vi "Sprinklernew.vi"() -> ()   [LabVIEW 2013]
doc: "This Vi is a simulation of Sprinkler system which service four zone\n-East\n-West\n-North\n-South\nIndicator on front panel indicate the zone that is currently running.\n\nThe controller loads the data to Zone Setup Array from .csv file.\n-It runs when user press start.\nWhen Run selector is at \nSingle position: the controller will serve each zone for the set timing and wait for input.\nContinuous Position: It will run contineously.\n\nSequence of operation: \nStart(Application): It will initialize all the controls and indicator to its default value.\nSetup: It will allow the user to change in Zone setup array.\nStart: It will start the VI.\nRain Sensor: Shows Rain in Status and indicators will not respond in this case."
uses:
  Controls/Sprinkler Cmd data cluster.ctl
  Controls/Sprinkler States.ctl
  SubVIs/water pressuer sensor fgv.ctl
  Controls/Read States.ctl
panel:
  in  "Zone Setup Array":cluster{"Zone Selector":string, "Timing":dbl}[](array[cluster])
  out "Controller Status":string
  out "Zone Indicators":T1
  in  "Water Pressure Sensor (%)":u32(slide) scale=0.0..100.0
  in  "Rain Sensor":bool
  in  "Run Selector":bool
  in  "Setup":bool
  in  "Start":bool
  in  "stop":bool
  # "Controls"
  # "Simulation Controls"
  # "Rain"
  # "No Rain"
  # "Continuous"
  # "Single"
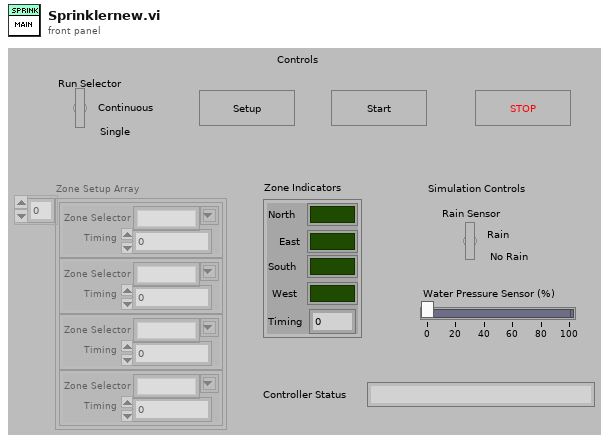
[diagram p1: front panel]
types:
  T1 = cluster{"North":bool, "East":bool, "South":bool, "West":bool, "Timing":u32}
  T2 = typedef "Sprinkler Cmd data cluster.ctl" = cluster{"Data":variant, "Command":T3}
  T3 = typedef "Sprinkler States.ctl" = enum16{"Initialize", "Setup", "Start", "Rain Sensor", "Stop"}
  T4 = typedef "water pressuer sensor fgv.ctl" = enum16{"Set data ", "Get data"}
  T5 = enum8{"Enabled", "Disabled", "Disabled and Grayed Out"}
  T6 = typedef "Read States.ctl" = enum16{"Initialize ", "Read", "Stop"}
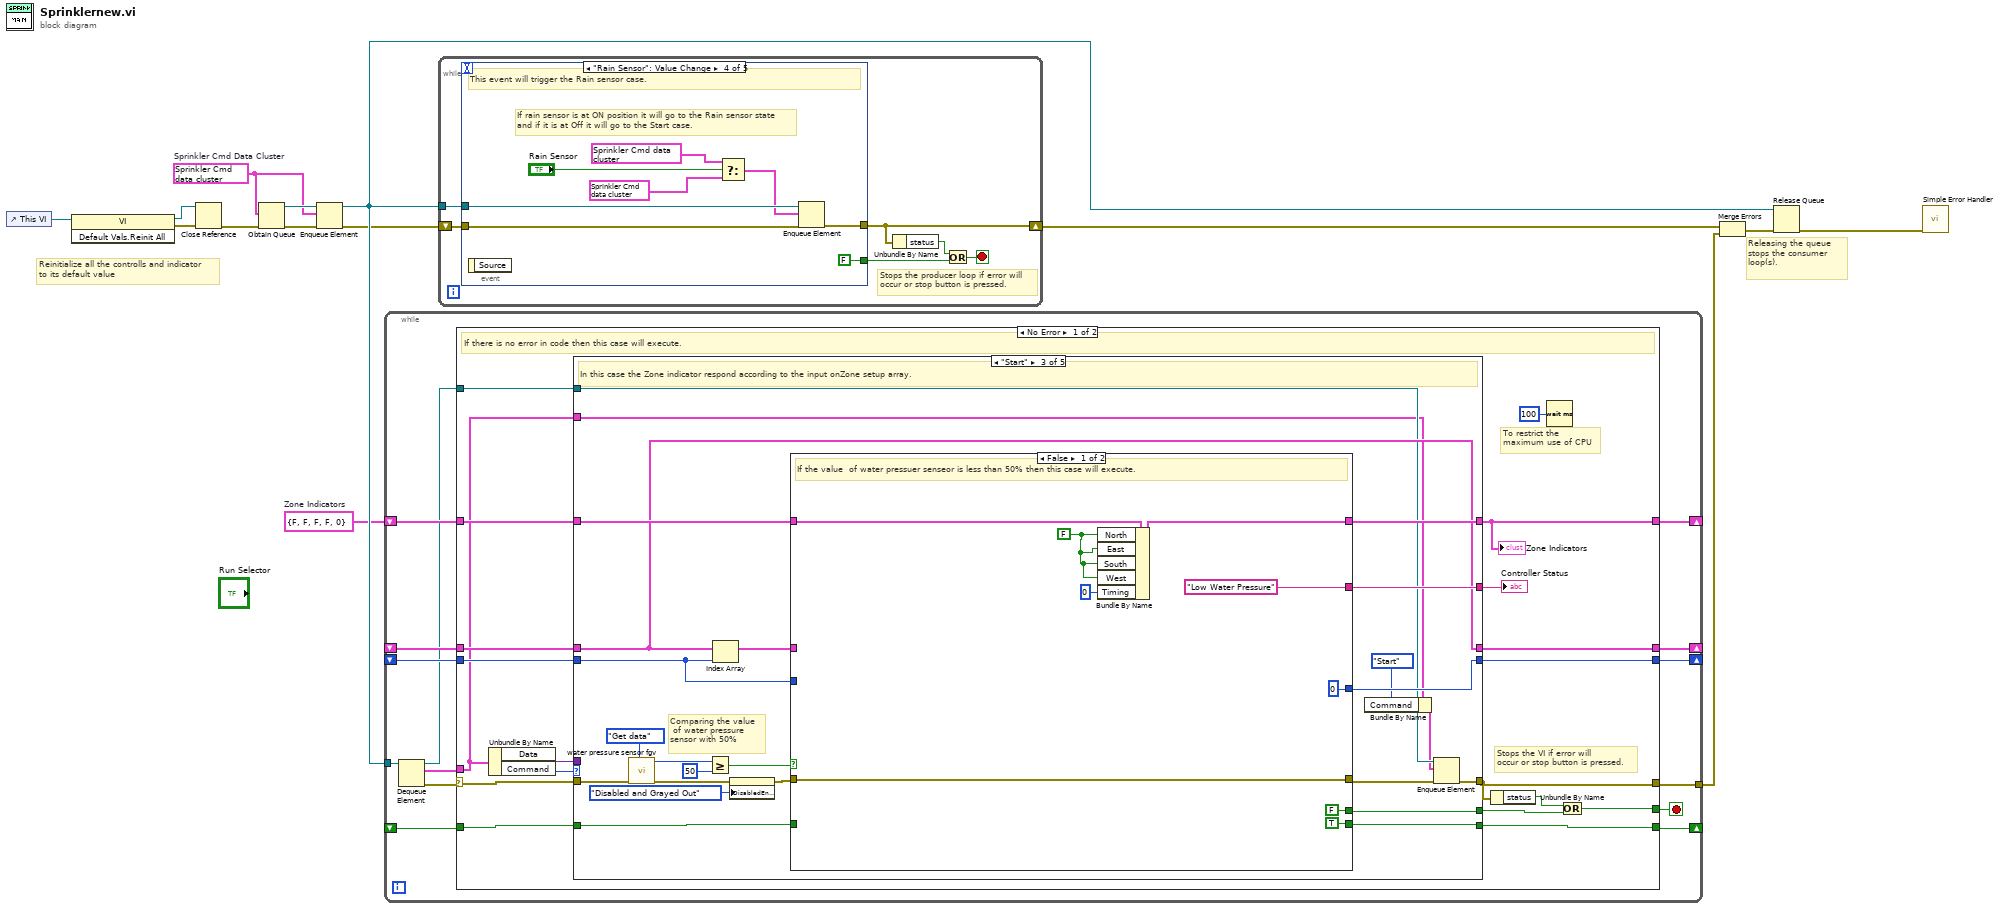
[diagram p0: block diagram]
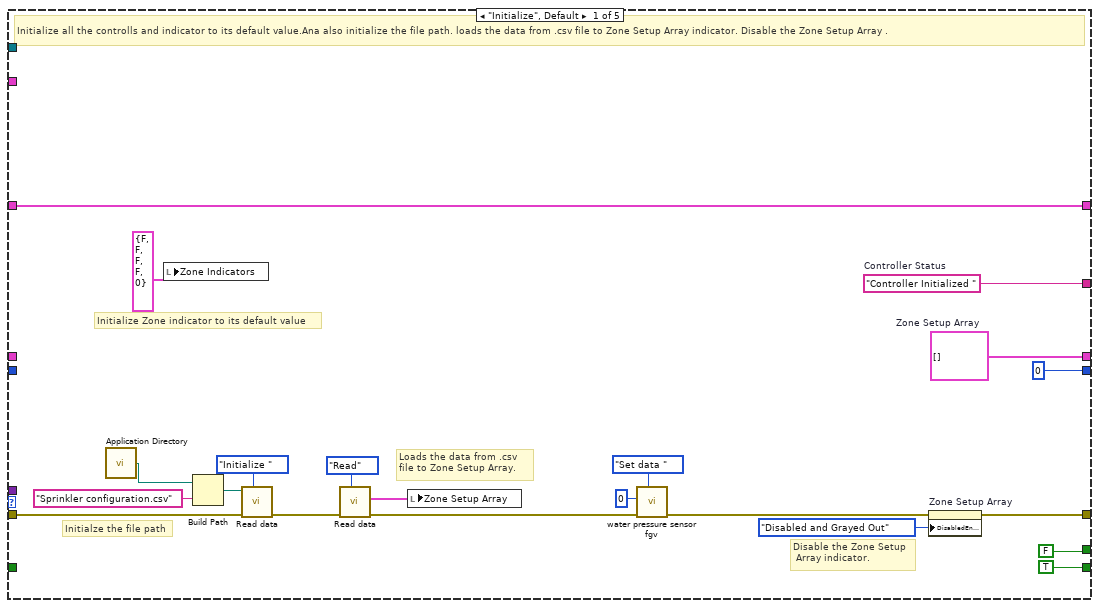
[diagram p2: hidden frame]
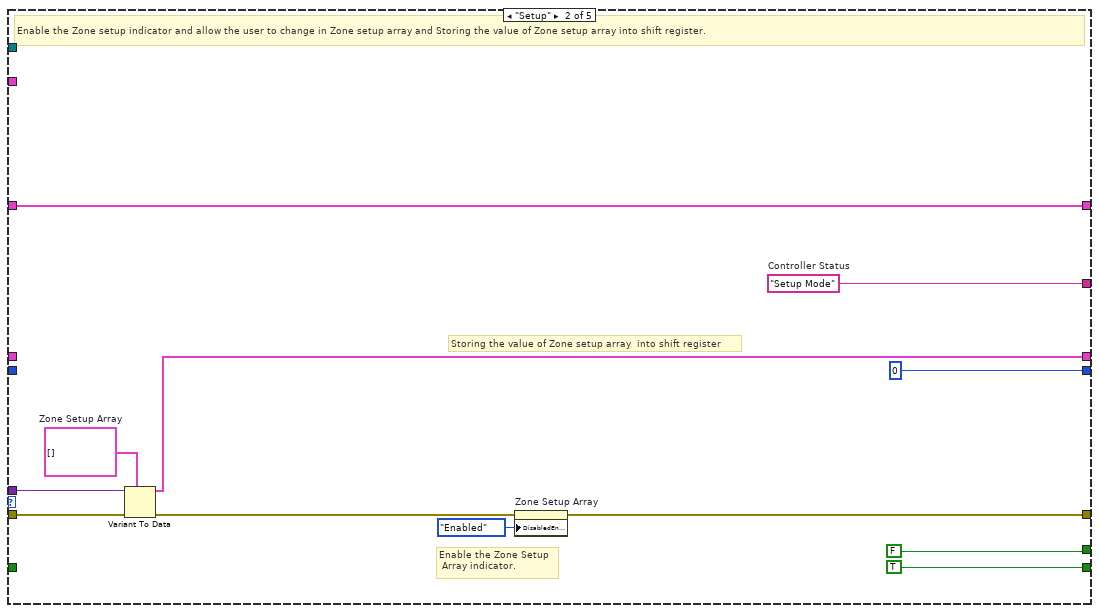
[diagram p3: hidden frame]
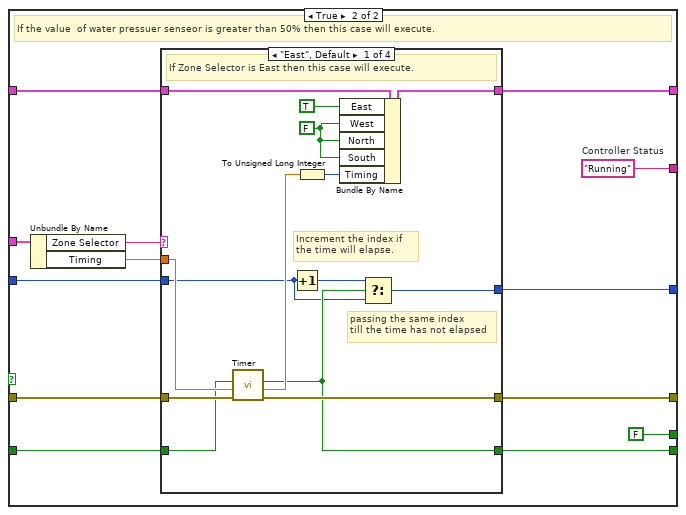
[diagram p4: hidden frame]
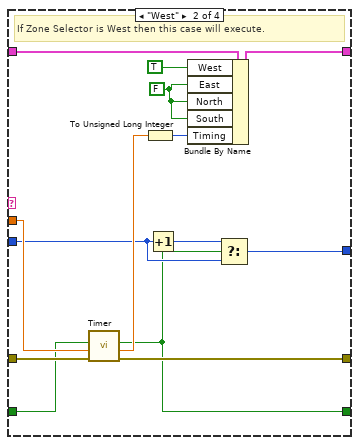
[diagram p5: hidden frame]
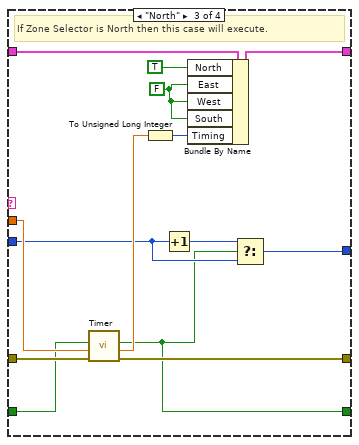
[diagram p6: hidden frame]
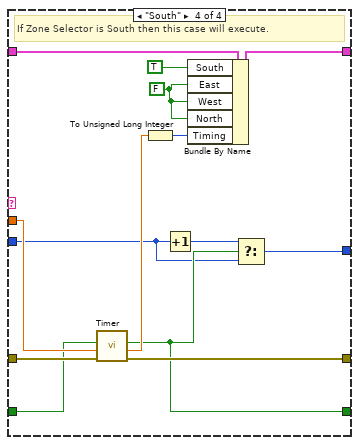
[diagram p7: hidden frame]
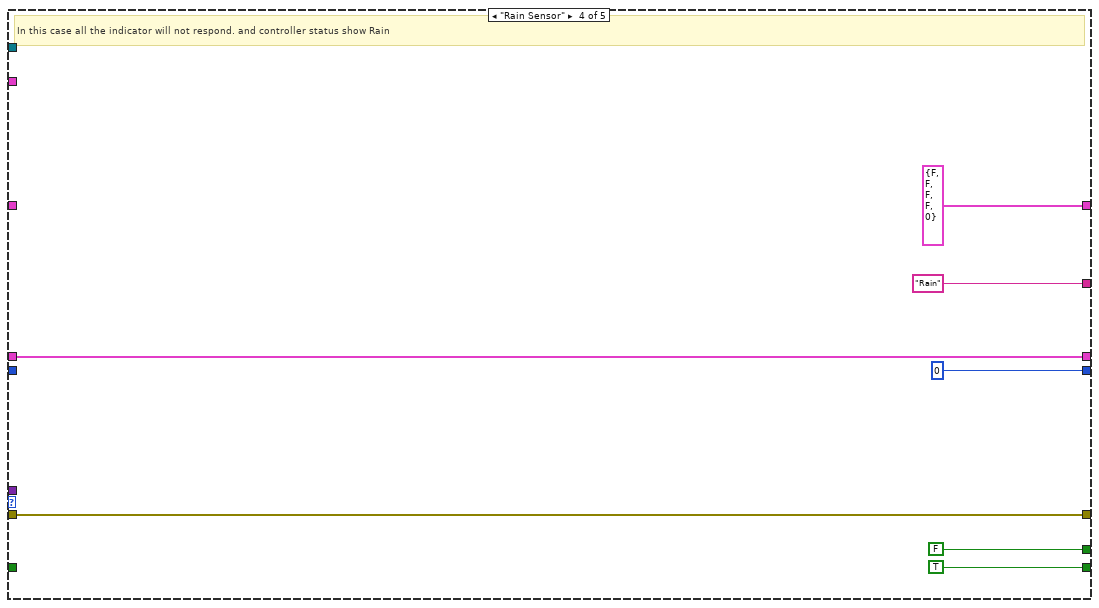
[diagram p8: hidden frame]
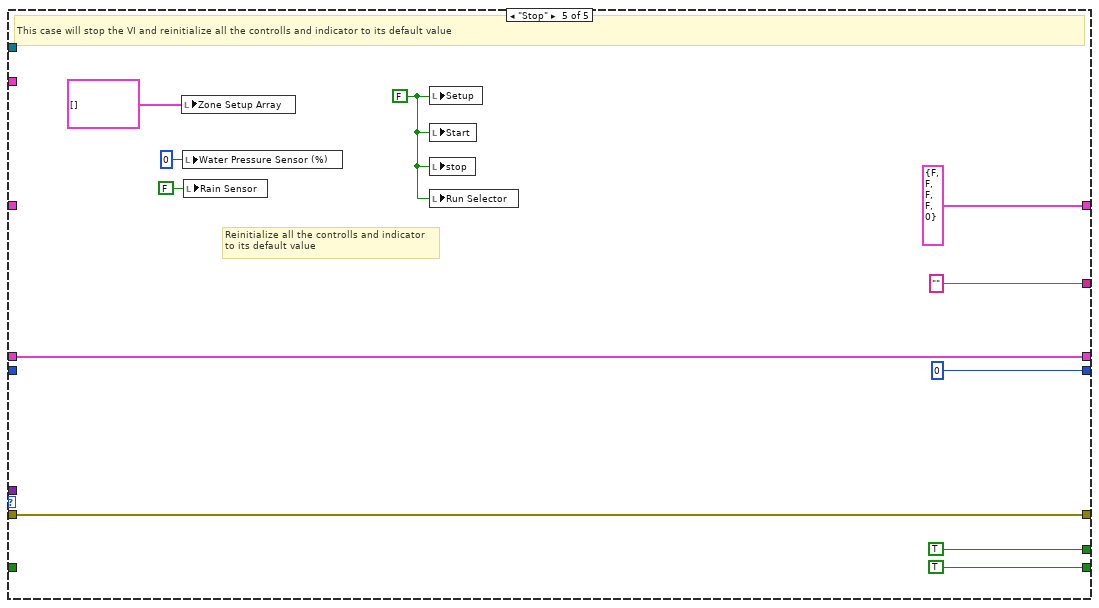
[diagram p9: hidden frame]
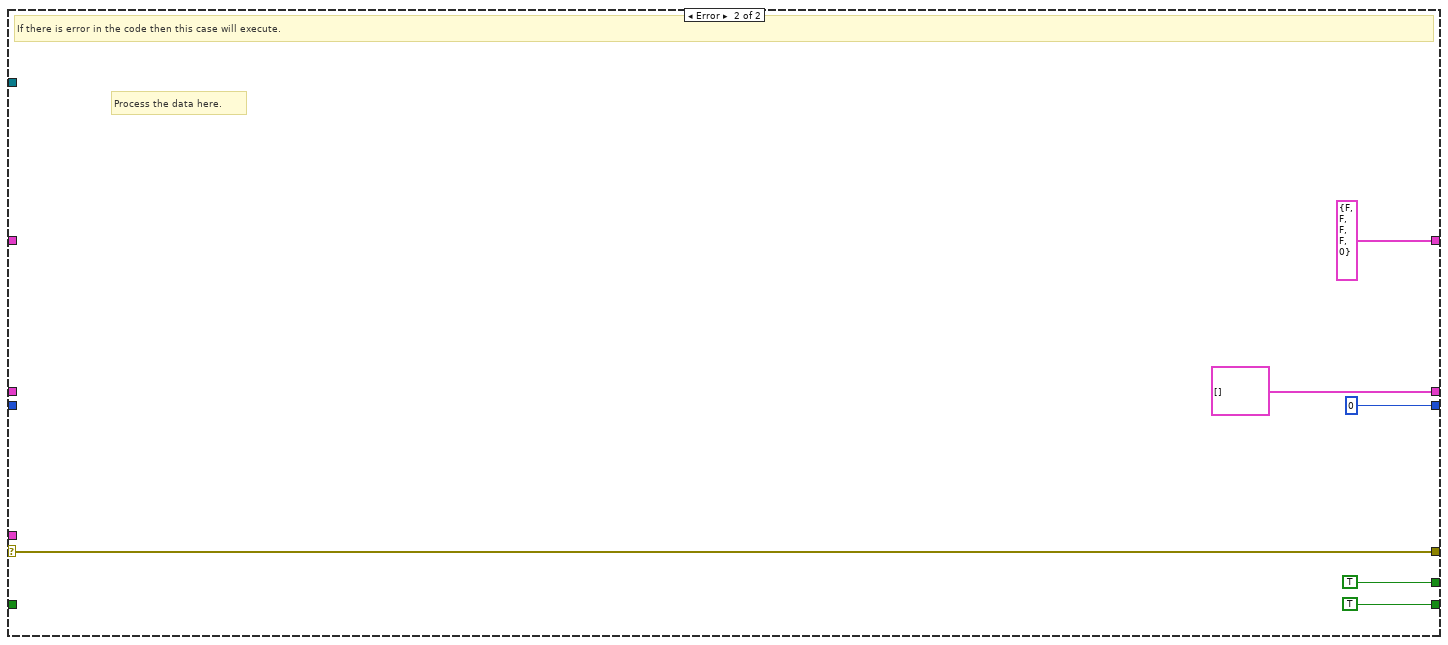
[diagram p10: hidden frame]
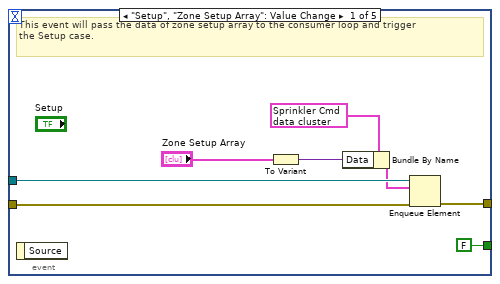
[diagram p11: hidden frame]
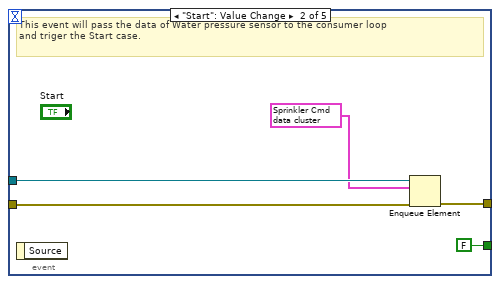
[diagram p12: hidden frame]
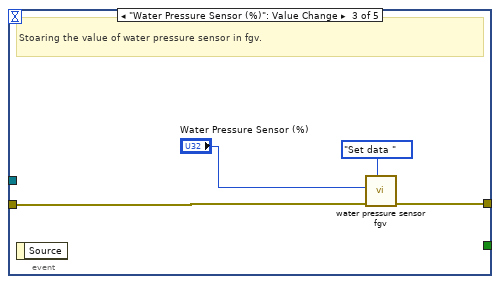
[diagram p13: hidden frame]
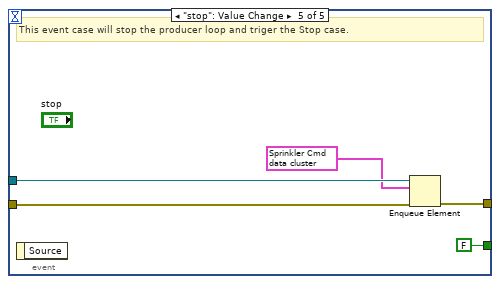
[diagram p14: hidden frame]
diagram:
  w1 = T1 {"North"=FALSE, "East"=FALSE, "South"=FALSE, "West"=FALSE, "Timing"=0}  # Zone Indicators
  w2 = T2 {"Data"=variant, "Command"=enum."Initialize"}  # Sprinkler Cmd Data Cluster
  # "Reinitialize all the controlls and indicator\nto its default value"
  # "Releasing the queue stops the consumer loop(s)."
  n1 = control-ref of="This VI"() -> (w10:refnum<vi>)
  n2 = invoke class="VI" method="Default Vals.Reinit All"(reference=w10) -> (reference out=w8:refnum<vi>, error out=w9:errorcluster)  [unwired: 2 in, 1 out]
  n3 = Close Reference(reference=w8, error in (no error)=w9) -> (error out=w3:errorcluster)
  n4 = Obtain Queue(element data type=w2, error in (no error)=w3) -> (queue out=w7:refnum<queue>, error out=w5:errorcluster)  [unwired: 3 in, 1 out]
  n5 = Enqueue Element(queue=w7, element=w2, error in (no error)=w5) -> (queue out=w6:refnum<queue>, error out=w4:errorcluster)  [unwired: 1 in, 1 out]
  n6 = while {
    tunnel: w6 -> [w28]
    tunnel: [w25] -> w12
    shift-right: [w23] -> _
    shift-left: w1 -> [w22]
    shift-right: [w21] -> _
    shift-left: _ -> [w20]
    shift-right: [w19] -> _
    shift-left: _ -> [w18]
    shift-right: [w17] -> _
    shift-left: _ -> [w16]
    stop <- w24 stop-if-true
    n7 = Dequeue Element(queue=w28) -> (queue out=w15:refnum<queue>, element=w26:T2, error out=w27:errorcluster)  [unwired: 2 in, 1 out]
    n8 = case shown="No Error" w27 {
      selector: w27 -> [w47 w205]
      tunnel: w26 -> [w29 _]
      tunnel: [w44 w205] -> w25
      tunnel: [w41 TRUE] -> w24
      tunnel: [w38 T1 {"North"=FALSE, "East"=FALSE, "South"=FALSE, "West"=FALSE, "Timing"=0} ("Zone Indicators")] -> w23
      tunnel: w22 -> [w39 _]
      tunnel: [w37 TRUE ("Boolean")] -> w21
      tunnel: w20 -> [w36 _]
      tunnel: [w35 cluster{"Zone Selector":string, "Timing":dbl}[] [] ("Zone Setup Array")] -> w19
      tunnel: w18 -> [w34 _]
      tunnel: [w33 0] -> w17
      tunnel: w16 -> [w32 _]
      tunnel: w15 -> [w30 _]
      frame No Error {
        # "Stops the VI if error will\noccur or stop button is pressed."
        # "To restrict the \nmaximum use of CPU"
        # "If there is no error in code then this case will execute."
        n9 = Unbundle By Name(w29) -> ("Data"=w40:variant, "Command"=w46:T3)
        n10 = case shown="\"Start\"" w46 {
          tunnel: [w60 w80 w86 w185 w196] -> w44
          tunnel: w47 -> [w67 w70 w90 w185 w196]
          tunnel: [w58 w78 w104 "Rain" ("Controller Status") "" ("Controller Status")] -> w45
          tunnel: [FALSE FALSE w103 FALSE TRUE] -> w42
          tunnel: w40 -> [_ w74 _ _ _]
          tunnel: [w54 w75 w98 T1 {"North"=FALSE, "East"=FALSE, "South"=FALSE, "West"=FALSE, "Timing"=0} ("Zone Indicators") T1 {"North"=FALSE, "East"=FALSE, "South"=FALSE, "West"=FALSE, "Timing"=0} ("Zone Indicators")] -> w38
          tunnel: w39 -> [w54 w75 w97 _ _]
          tunnel: [TRUE ("Boolean") TRUE w95 TRUE ("Elapsed?") TRUE ("Elapsed?")] -> w37
          tunnel: w36 -> [_ _ w96 _ _]
          tunnel: [w53 w73 w93 w187 w198] -> w35
          tunnel: w34 -> [_ _ w93 w187 w198]
          tunnel: [0 0 w91 0 0] -> w33
          tunnel: w32 -> [_ _ w92 _ _]
          tunnel: w30 -> [_ _ w85 _ _]
          tunnel: w29 -> [_ _ w84 _ _]
          frame "Initialize", Default {
            w53 = cluster{"Zone Selector":string, "Timing":dbl}[] []  # Zone Setup Array
            w58 = "Controller Initialized "  # Controller Status
            # "Disable the Zone Setup\n Array indicator."
            # "Loads the data from .csv \nfile to Zone Setup Array."
            # "Initialze the file path"
            # "Initialize Zone indicator to its default value"
            # "Initialize all the controlls and indicator to its default value.Ana also initialize the file path. loads the data from .csv file to Zone Setup Array indicator. Disable the Zone Setup Array ."
            n11 = call <vilib>:"Application Directory.vi"() -> ("Application Directory"=w66:path)
            n12 = local write "Zone Indicators"(T1 {"North"=FALSE, "East"=FALSE, "South"=FALSE, "West"=FALSE, "Timing"=0} ("Zone Indicators")) -> ()
            n13 = Build Path(base path=w66, name or relative path="Sprinkler configuration.csv") -> (appended path=w65:path)
            n14 = call "Read data.vi"("Command"=Read_States."Initialize ", "error in"=w67, "file path"=w65) -> ("error out"=w63:errorcluster)  [unwired: 7 in, 1 out]
            n15 = call "Read data.vi"("Command"=Read_States."Read", "error in"=w63) -> ("error out"=w51:errorcluster, "Zone Setup Array"=w61:cluster{string, dbl}[])  [unwired: 8 in]
            n16 = local write "Zone Setup Array"(w61) -> ()
            n17 = call "water pressure sensor fgv.vi"("Command"=water_pressuer_sensor_fgv."Set data ", "error constant"=w51, "Sprinkler Cmd Data Cluster"=u32 0) -> ("error IO"=w50:errorcluster)  [unwired: 7 in, 1 out]
            n18 = property on="Zone Setup Array" class="Arr (strict)"(error in=w50, "DisabledEnum"=T5."Disabled and Grayed Out" ("Disabled")) -> (error out=w60:errorcluster)  [unwired: 1 in, 1 out]
          }
          frame "Setup" {
            w72 = cluster{"Zone Selector":string, "Timing":dbl}[] []  # Zone Setup Array
            w78 = "Setup Mode"  # Controller Status
            # "Storing the value of Zone setup array  into shift register"
            # "Enable the Zone Setup\n Array indicator."
            # "Enable the Zone setup indicator and allow the user to change in Zone setup array and Storing the value of Zone setup array into shift register."
            n19 = Variant To Data(error in=w70, type=w72, Variant=w74) -> (data=w73:cluster{"Zone Selector":string, "Timing":dbl}[], error out=w69:errorcluster)
            n20 = property on="Zone Setup Array" class="Arr (strict)"(error in=w69, "DisabledEnum"=T5."Enabled" ("Disabled")) -> (error out=w80:errorcluster)  [unwired: 1 in, 1 out]
          }
          frame "Start" {
            # "Comparing the value\n of water pressure \nsensor with 50%"
            # "In this case the Zone indicator respond according to the input onZone setup array."
            n21 = call "water pressure sensor fgv.vi"("Command"=water_pressuer_sensor_fgv."Get data", "error constant"=w90) -> ("error IO"=w89:errorcluster, "Sprinkler Cmd Data Cluster"=w88:u32)  [unwired: 8 in]
            n22 = Greater Or Equal?(x=w88, y=u32 50) -> (x >= y?=w101:bool)
            n23 = Index Array "Index Array"(array=w93, index=w92) -> (element=w94:cluster{"Zone Selector":string, "Timing":dbl})
            n24 = property on="Zone Setup Array" class="Arr (strict)"(error in=w89, "DisabledEnum"=T5."Disabled and Grayed Out" ("Disabled")) -> (error out=w99:errorcluster)  [unwired: 1 in, 1 out]
            n25 = case shown="False" w101 {
              tunnel: ["Low Water Pressure" ("Controller Status") w126] -> w104
              tunnel: [FALSE FALSE] -> w103
              tunnel: w99 -> [w112 w124]
              tunnel: [w112 w123] -> w87
              tunnel: w94 -> [_ w122]
              tunnel: [w107 w120] -> w98
              tunnel: w97 -> [w111 w119]
              tunnel: w96 -> [_ w117]
              tunnel: [TRUE ("Boolean") w116] -> w95
              tunnel: w92 -> [_ w115]
              tunnel: [0 w114] -> w91
              frame False {
                w105 = FALSE ("North")
                # "If the value  of water pressuer senseor is less than 50% then this case will execute."
                n26 = Bundle By Name(cluster=w111, "North"=w105, "East"=w105, "South"=w105, "West"=w105, "Timing"=u32 0) -> (w107:T1)
              }
              frame True {
                w126 = "Running"  # Controller Status
                # "If the value  of water pressuer senseor is greater than 50% then this case will execute."
                n27 = Unbundle By Name(w122) -> ("Zone Selector"=w121:string, "Timing"=w118:dbl)
                n28 = case shown="\"East\", Default" w121 {
                  tunnel: w124 -> [w137 w151 w165 w179]
                  tunnel: [w136 w150 w164 w178] -> w123
                  tunnel: [w139 w153 w167 w181] -> w120
                  tunnel: w119 -> [w140 w154 w168 w182]
                  tunnel: w118 -> [w135 w149 w163 w177]
                  tunnel: w117 -> [w134 w148 w162 w176]
                  tunnel: [w130 w142 w155 w170] -> w116
                  tunnel: w115 -> [w128 w143 w156 w169]
                  tunnel: [w127 w141 w157 w171] -> w114
                  frame "East", Default {
                    w131 = FALSE
                    # "passing the same index \ntill the time has not elapsed"
                    # "Increment the index if \nthe time will elapse."
                    # "If Zone Selector is East then this case will execute."
                    n29 = call "Timer.vi"("error in (no error)"=w137, "Time Target(s)"=w135, "Reset"=w134) -> ("error out"=w136:errorcluster, "Elapsed Time"=w133:dbl, "Elapsed?"=w130:bool)  [unwired: 6 in]
                    n30 = Increment(x=w128) -> (x+1=w129:i32)
                    n31 = To Unsigned Long Integer(number=w133) -> (unsigned 32bit integer=w132:u32)
                    n32 = Bundle By Name(cluster=w140, "East"=TRUE, "West"=w131, "North"=w131, "South"=w131, "Timing"=w132) -> (w139:T1)
                    n33 = Select(t=w129, s=w130, f=w128) -> (s? t:f=w127:i32)
                  }
                  frame "West" {
                    w145 = FALSE
                    # "If Zone Selector is West then this case will execute."
                    n34 = call "Timer.vi"("error in (no error)"=w151, "Time Target(s)"=w149, "Reset"=w148) -> ("error out"=w150:errorcluster, "Elapsed Time"=w147:dbl, "Elapsed?"=w142:bool)  [unwired: 6 in]
                    n35 = To Unsigned Long Integer(number=w147) -> (unsigned 32bit integer=w146:u32)
                    n36 = Increment(x=w143) -> (x+1=w144:i32)
                    n37 = Bundle By Name(cluster=w154, "West"=TRUE ("East"), "East"=w145, "North"=w145, "South"=w145, "Timing"=w146) -> (w153:T1)
                    n38 = Select(t=w144, s=w142, f=w143) -> (s? t:f=w141:i32)
                  }
                  frame "North" {
                    w159 = FALSE
                    # "If Zone Selector is North then this case will execute."
                    n39 = call "Timer.vi"("error in (no error)"=w165, "Time Target(s)"=w163, "Reset"=w162) -> ("error out"=w164:errorcluster, "Elapsed Time"=w161:dbl, "Elapsed?"=w155:bool)  [unwired: 6 in]
                    n40 = To Unsigned Long Integer(number=w161) -> (unsigned 32bit integer=w160:u32)
                    n41 = Increment(x=w156) -> (x+1=w158:i32)
                    n42 = Bundle By Name(cluster=w168, "North"=TRUE ("East"), "East"=w159, "West"=w159, "South"=w159, "Timing"=w160) -> (w167:T1)
                    n43 = Select(t=w158, s=w155, f=w156) -> (s? t:f=w157:i32)
                  }
                  frame "South" {
                    w173 = FALSE
                    # "If Zone Selector is South then this case will execute."
                    n44 = call "Timer.vi"("error in (no error)"=w179, "Time Target(s)"=w177, "Reset"=w176) -> ("error out"=w178:errorcluster, "Elapsed Time"=w175:dbl, "Elapsed?"=w170:bool)  [unwired: 6 in]
                    n45 = To Unsigned Long Integer(number=w175) -> (unsigned 32bit integer=w174:u32)
                    n46 = Increment(x=w169) -> (x+1=w172:i32)
                    n47 = Bundle By Name(cluster=w182, "South"=TRUE ("East"), "East"=w173, "West"=w173, "North"=w173, "Timing"=w174) -> (w181:T1)
                    n48 = Select(t=w172, s=w170, f=w169) -> (s? t:f=w171:i32)
                  }
                }
              }
            }
            n49 = Bundle By Name(cluster=w84, "Command"=Sprinkler_States."Start") -> (w83:T2)
            n50 = Enqueue Element(queue=w85, element=w83, error in (no error)=w87) -> (error out=w86:errorcluster)  [unwired: 1 in, 2 out]
          }
          frame "Rain Sensor" {
            # "In this case all the indicator will not respond. and controller status show Rain"
          }
          frame "Stop" {
            w190 = FALSE
            # "Reinitialize all the controlls and indicator\nto its default value"
            # "This case will stop the VI and reinitialize all the controlls and indicator to its default value"
            n51 = local write "Zone Setup Array"(cluster{"Zone Selector":string, "Timing":dbl}[] [] ("Zone Setup Array")) -> ()
            n52 = local write "Water Pressure Sensor (%)"(u32 0 ("Water Pressure Sensor (%)")) -> ()
            n53 = local write "Rain Sensor"(FALSE ("Rain Sensor")) -> ()
            n54 = local write "Setup"(w190) -> ()
            n55 = local write "Start"(w190) -> ()
            n56 = local write "stop"(w190) -> ()
            n57 = local write "Run Selector"(w190) -> ()
          }
        }
        "Controller Status" <- w45
        "Zone Indicators" <- w38
        n58 = Unbundle By Name(w44) -> ("status"=w43:bool)
        n59 = Wait (ms)(milliseconds to wait=u32 100) -> ()  [unwired: 1 out]
        n60 = Or(x=w43, y=w42) -> (x .or. y?=w41:bool)
      }
      frame Error {
        # "Process the data here."
        # "If there is error in the code then this case will execute."
      }
    }
  }
  n61 = while {
    shift-right: [w209] -> w14
    shift-left: w4 -> [w211]
    tunnel: w6 -> [w212]
    stop <- w210 stop-if-true
    # "Stops the producer loop if error will\noccur or stop button is pressed."
    n62 = event shown="[3] \"Rain Sensor\": Value Change" {
      selector: _ -> [_ _ _ _ _]
      dyn-events: _ -> [_ _ _ _ _]
      timeout: _ -> [_ _ _ _ _]
      tunnel: w212 -> [w220 w225 _ w237 w242]
      tunnel: w211 -> [w219 w224 w229 w236 w241]
      tunnel: [w218 w223 w228 w235 w240] -> w209
      tunnel: [FALSE FALSE _ FALSE FALSE] -> w207
      event "Setup", "Zone Setup Array": Value Change {
        # "This event will pass the data of zone setup array to the consumer loop and trigger \nthe Setup case."
        n63 = event-data() -> ()  [unwired: 1 in, 1 out]
        n64 = To Variant(anything="Zone Setup Array") -> (Variant=w213:variant)
        n65 = Bundle By Name(cluster=T2 {"Data"=variant, "Command"=enum."Setup"} ("Sprinkler Cmd Data Cluster"), "Data"=w213) -> (w215:T2)
        n66 = Enqueue Element(queue=w220, element=w215, error in (no error)=w219) -> (error out=w218:errorcluster)  [unwired: 1 in, 2 out]
      }
      event "Start": Value Change {
        # "This event will pass the data of Water pressure sensor to the consumer loop\nand triger the Start case."
        n67 = event-data() -> ()  [unwired: 1 in, 1 out]
        n68 = Enqueue Element(queue=w225, element=T2 {"Data"=variant, "Command"=enum."Start"} ("Sprinkler Cmd Data Cluster"), error in (no error)=w224) -> (error out=w223:errorcluster)  [unwired: 1 in, 2 out]
      }
      event "Water Pressure Sensor (%)": Value Change {
        # "Stoaring the value of water pressure sensor in fgv."
        n69 = event-data() -> ()  [unwired: 1 in, 1 out]
        n70 = call "water pressure sensor fgv.vi"("Command"=water_pressuer_sensor_fgv."Set data ", "error constant"=w229, "Sprinkler Cmd Data Cluster"="Water Pressure Sensor (%)") -> ("error IO"=w228:errorcluster)  [unwired: 7 in, 1 out]
      }
      event "Rain Sensor": Value Change {
        # "If rain sensor is at ON position it will go to the Rain sensor state\nand if it is at Off it will go to the Start case."
        # "This event will trigger the Rain sensor case."
        n71 = event-data() -> ()  [unwired: 1 in, 1 out]
        n72 = Select(t=T2 {"Data"=variant, "Command"=enum."Rain Sensor"} ("Sprinkler Cmd Data Cluster"), s="Rain Sensor", f=T2 {"Data"=variant, "Command"=enum."Start"} ("Sprinkler Cmd Data Cluster")) -> (s? t:f=w230:T2)
        n73 = Enqueue Element(queue=w237, element=w230, error in (no error)=w236) -> (error out=w235:errorcluster)  [unwired: 1 in, 2 out]
      }
      event "stop": Value Change {
        # "This event case will stop the producer loop and triger the Stop case."
        n74 = event-data() -> ()  [unwired: 1 in, 1 out]
        n75 = Enqueue Element(queue=w242, element=T2 {"Data"=variant, "Command"=enum."Stop"} ("Sprinkler Cmd Data Cluster"), error in (no error)=w241) -> (error out=w240:errorcluster)  [unwired: 1 in, 2 out]
      }
    }
    n76 = Unbundle By Name(w209) -> ("status"=w208:bool)
    n77 = Or(x=w208, y=w207) -> (x .or. y?=w210:bool)
  }
  n78 = Merge Errors(w14, w12) -> (w13:errorcluster)
  n79 = Release Queue(queue=w6, error in (no error)=w13) -> (error out=w11:errorcluster)  [unwired: 1 in, 2 out]
  n80 = call <vilib>:"Simple Error Handler.vi"("error in (no error)"=w11) -> ()  [unwired: 4 in, 5 out]
